vi "Day-01 pt 2 Sonar Sweep Moving Average.vi"() -> ()   [LabVIEW 2020, in "Advent of Code.lvlib"]
uses:
  Advent of Code.lvlib
panel:
  out "# of increases":i32
  in  "Input":string
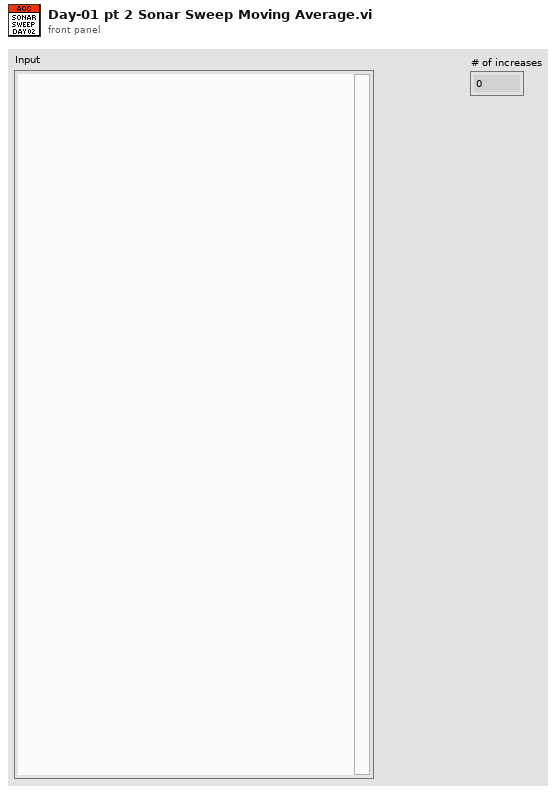
[diagram p1: front panel]
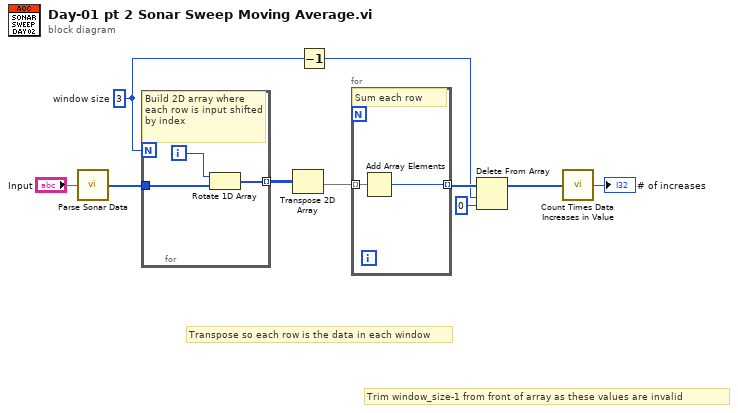
[diagram p0: block diagram]
diagram:
  w6 = 3  # window size
  # "Trim window_size-1 from front of array as these values are invalid"
  # "Transpose so each row is the data in each window"
  n1 = call "Parse Sonar Data.vi"("Sonar Values String"="Input") -> ("Sonar Data"=w1:i32[])
  n2 = for {
    N: w6 -> [_]
    tunnel: w1 -> [w13]
    tunnel: [w11] -> w9 mode=indexing
    i -> [w12]
    # "Build 2D array where each row is input shifted by index"
    n3 = Rotate 1D Array(1:w13, 2:w12) -> (0:w11:i32[])
  }
  n4 = Transpose 2D Array(2D array=w9) -> (transposed array=w8:i32[][])
  n5 = Decrement(x=w6) -> (x-1=w5:i32)
  n6 = for {
    tunnel: w8 -> [w15] mode=indexing
    tunnel: [w14] -> w7 mode=indexing
    # "Sum each row"
    n7 = Add Array Elements(numeric array=w15) -> (sum=w14:i32)
  }
  n8 = Delete From Array(array=w7, length=w5, index=0) -> (array with subset deleted=w3:i32[])  [unwired: 1 out]
  n9 = call "Count Times Data Increases in Value.vi"("Data"=w3) -> ("Count Increases"=→"# of increases":i32)
